vi "InitiateClientHandshake.vi"(6 "WS URI":string="ws://hostname.domain:80/resource/name", 7 "additional headers (none)":T1[](array[typedef]), 8 "error in (no error)":errorcluster, 9 "timeout ms (5000)":i32=5000, 10 "Relative URI Request (F)":bool, 11 "WebSocket Connection in":refnum<k5>) -> (0 "error out":errorcluster, 2 "Return Headers Out":variant, 3 "WebSocket Connection out":refnum<k5>)   [LabVIEW 2016, in "WebSockets.lvlib"]
doc: "Performs a client-side handshake. Sends the initial handshake HTTP header and waits for response from WebSocket server. Validates received accept key from the response.\nWebSockets 1.6.0.22\nSam Sharp - MediaMongrels Ltd\nCopyright (c) 2016, MediaMongrels Ltd"
uses:
  WebSockets.lvlib
  Headers.ctl
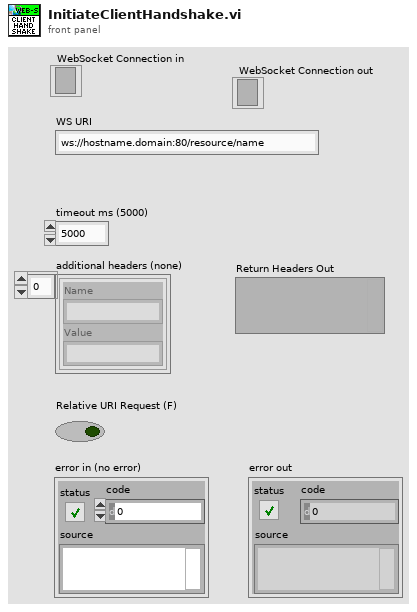
[diagram p1: front panel]
types:
  T1 = typedef "WebSockets.lvlib/Headers.ctl" = cluster{"Name":string, "Value":string}
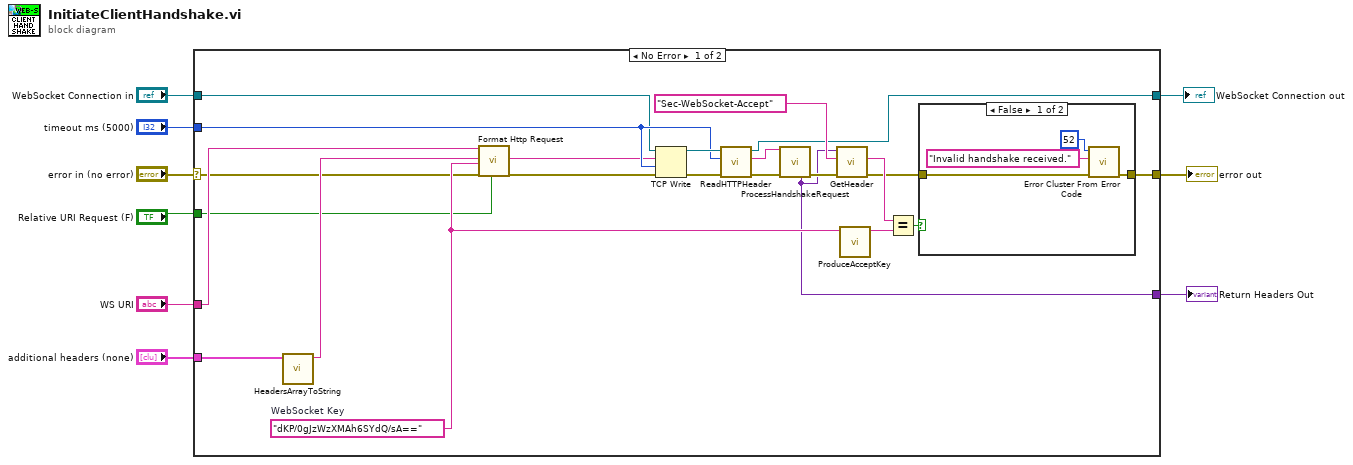
[diagram p0: block diagram]
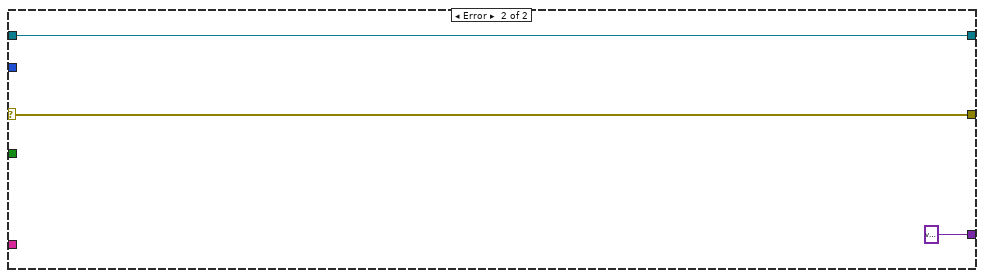
[diagram p3: hidden frame]
diagram:
  n1 = case shown="No Error" "error in (no error)" {
    selector: "error in (no error)" -> [w13 w40]
    tunnel: [w21 w39] -> w9
    tunnel: "WebSocket Connection in" -> [w17 w39]
    tunnel: [w18 w40] -> w6
    tunnel: "timeout ms (5000)" -> [w30 _]
    tunnel: [w23 variant ("Headers Out")] -> w4
    tunnel: "WS URI" -> [w14 _]
    tunnel: "additional headers (none)" -> [w16 _]
    tunnel: "Relative URI Request (F)" -> [w10 _]
    frame No Error {
      w27 = "dKP/0gJzWzXMAh6SYdQ/sA=="  # WebSocket Key
      n2 = call "HeadersArrayToString.vi"("additional headers (none)"=w16) -> ("header string out"=w15:string)  [unwired: 10 in]
      n3 = call "Format Http Request.vi"("WS URI"=w14, "header string in"=w15, "WebSocket Key"=w27, "error in"=w13, "Relative URI Request (F)"=w10) -> ("Http Request"=w11:string, "error out"=w12:errorcluster)  [unwired: 13 in]
      n4 = TCP Write(connection ID=w17, data in=w11, error in (no error)=w12, 9:w30) -> (connection ID out=w31:refnum<k5>, error out=w32:errorcluster)  [unwired: 1 out]
      n5 = call "ReadHTTPHeader.vi"("error in (no error)"=w32, "timeout ms (25000)"=w30, "WebSocket Connection in"=w31) -> ("error out"=w22:errorcluster, "HTTP Header"=w28:string, "WebSocket Connection out"=w21:refnum<k5>)  [unwired: 6 in]
      n6 = call "ProcessHandshakeRequest.vi"("HTTP Headers"=w28, "error in (no error)"=w22) -> ("Headers Out"=w23:variant, "error out"=w26:errorcluster)  [unwired: 7 in, 5 out]
      n7 = call "GetHeader.vi"("error in (no error)"=w26, "Name"="Sec-WebSocket-Accept", "Headers In"=w23) -> ("error out"=w19:errorcluster, "Data"=w24:string)  [unwired: 5 in, 2 out]
      n8 = call "ProduceAcceptKey.vi"("Sec-WebSocket-Key"=w27) -> ("Sec-WebSocket-Accept"=w29:string)  [unwired: 10 in]
      n9 = Equal?(x=w24, y=w29) -> (x = y?=w20:bool)
      n10 = case shown="False" w20 {
        tunnel: w19 -> [w35 w37]
        tunnel: [w36 w37] -> w18
        frame False {
          n11 = call <vilib>:"Error Cluster From Error Code.vi"("error in (no error)"=w35, "error message (\"\")"="Invalid handshake received." ("error message (\"\")"), "error code (0)"=52) -> ("error out"=w36:errorcluster)  [unwired: 6 in]
        }
        frame True {
        }
      }
    }
    frame Error {
    }
  }
  "WebSocket Connection out" <- w9
  "error out" <- w6
  "Return Headers Out" <- w4
